vi "Inject Lookup Table.vi"(9 "LookupTable":refnum<data-value>, 11 "Process Model in":refnum<class "Process Model.lvclass">) -> (3 "Process Model out":refnum<class "Process Model.lvclass">)   [LabVIEW 2019, in "Test Executive.lvlib" / "Parallelizer Example.lvlib" / "Process Model.lvclass"]
uses:
  <vilib>/gpm_packages/@cs/test-executive/Source/Sandbox/Parallelizer Example/Process Model/Process Model.lvclass
  <vilib>/gpm_packages/@cs/lookup-table/Source/LookupTable/LookupTable.lvclass
  <vilib>/gpm_packages/@cs/test-executive/Source/Sandbox/Parallelizer Example/Process Model/Process Model.lvclass/Process Model.ctl
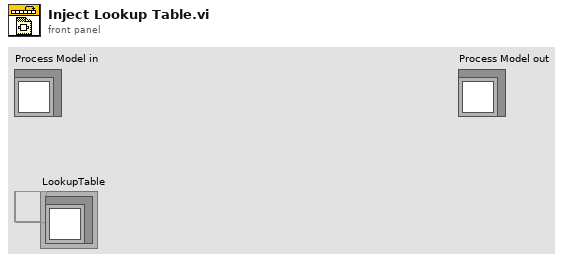
[diagram p1: front panel]
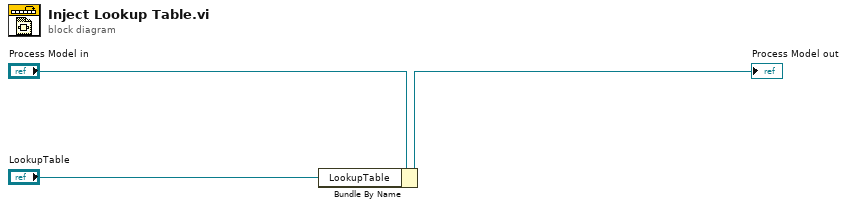
[diagram p0: block diagram]
diagram:
  n1 = Bundle By Name(cluster="Process Model in", "LookupTable"="LookupTable") -> (→"Process Model out":refnum<class "Process Model.lvclass">)
